vi "TCP Named Service - Server.vi"() -> ()   [LabVIEW 2019]
doc: "创建一个命名服务并在第一个可用端口侦听。当客户端连接该服务时，将发送一个响应字符串至客户端。"
panel:
  in  "服务器关闭":string="服务器VI关闭了连接。"
  in  "停止 2":bool
  out "波形图":dbl[](graph)
  # "概述：演示使用TCP函数初始化可向客户端VI发送数据的命名TCP服务。\n操作步骤:\n1.运行VI。\n2.打开TCP Named Service - Client.vi并按照前面板上的说明操作。\n3.单击停止 停止VI运行。"
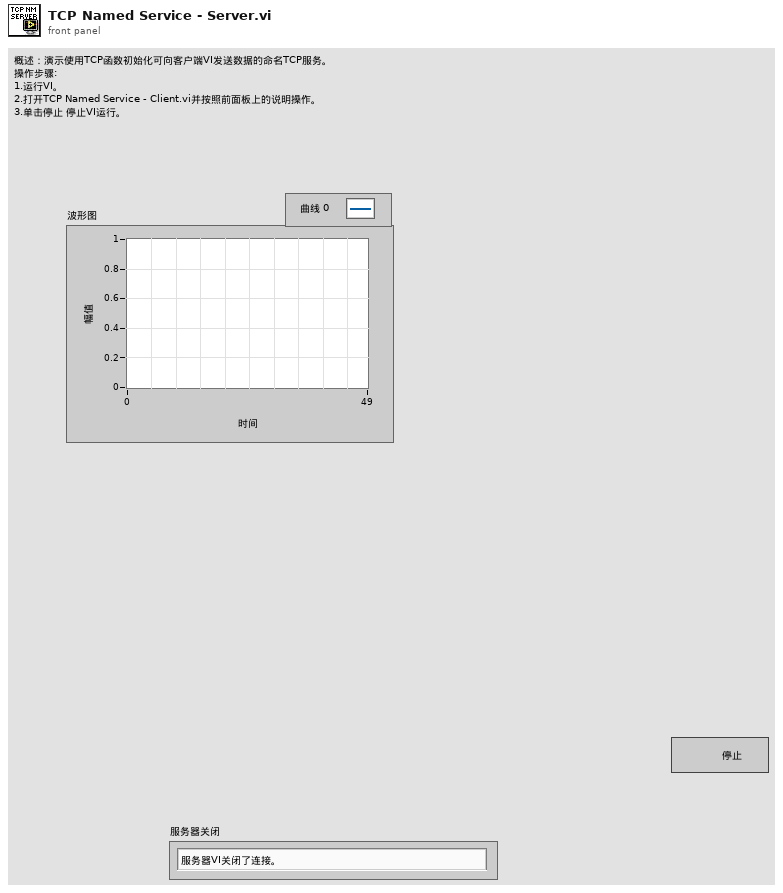
[diagram p1: front panel]
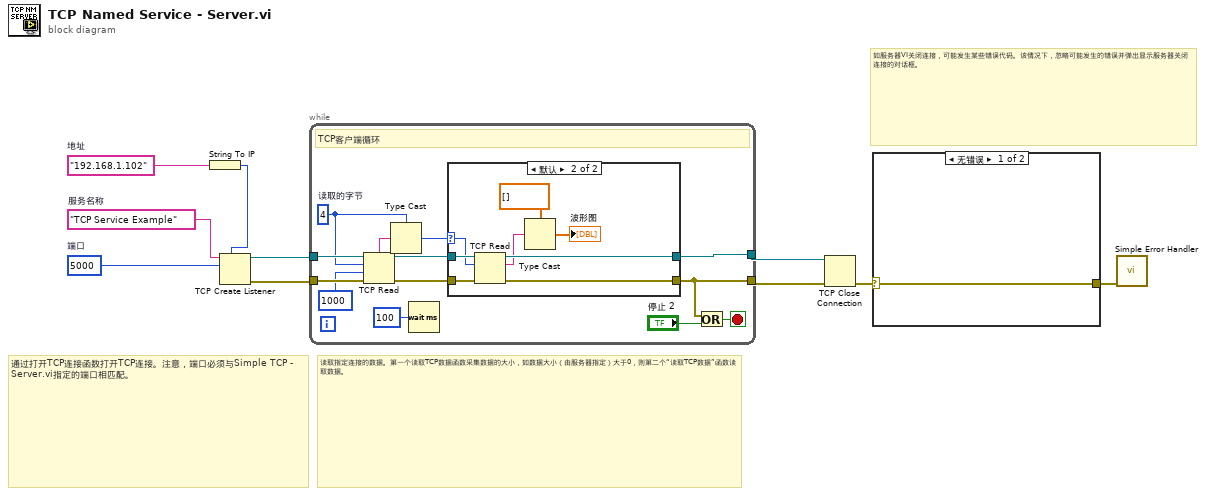
[diagram p0: block diagram]
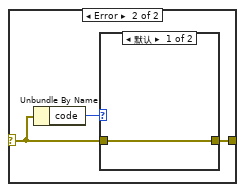
[diagram p2: hidden frame]
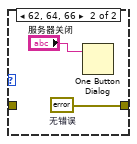
[diagram p3: hidden frame]
diagram:
  w6 = "192.168.1.102"  # 地址
  w8 = u16 5000  # 端口
  w7 = "TCP Service Example"  # 服务名称
  # "如服务器VI关闭连接，可能发生某些错误代码。该情况下，忽略可能发生的错误并弹出显示服务器关闭连接的对话框。"
  # "读取指定连接的数据。第一个读取TCP数据函数采集数据的大小，如数据大小（由服务器指定）大于0，则第二个“读取TCP数据”函数读取数据。"
  # "通过打开TCP连接函数打开TCP连接。注意，端口必须与Simple TCP - Server.vi指定的端口相匹配。"
  n1 = String To IP(1:w6) -> (0:w5:u32)
  n2 = TCP Create Listener(7:w5, 10:w8, 11:w7) -> (0:w3:errorcluster, 3:w4:refnum<k5>)  [unwired: 2 in, 1 out]
  n3 = while {
    tunnel: w3 -> [w19]
    tunnel: w4 -> [w20]
    tunnel: [w14] -> w2
    tunnel: [w13] -> w1
    stop <- w16 stop-if-true
    w18 = 4  # 读取的字节
    # "TCP客户端循环"
    n4 = TCP Read(connection ID=w20, bytes to read=w18, error in (no error)=w19, 9:1000 ("timeout ms (25000)")) -> (connection ID out=w22:refnum<k5>, data out=w23:string, error out=w21:errorcluster)  [unwired: 1 in]
    n5 = Type Cast(type=w18, x=w23) -> (*(type *) &x=w12:i32)
    n6 = Wait (ms)(milliseconds to wait=u32 100) -> ()  [unwired: 1 out]
    n7 = case shown="默认" w12 {
      selector: w12 -> [_ w26]
      tunnel: w22 -> [w25 w33]
      tunnel: w21 -> [w24 w32]
      tunnel: [w25 w29] -> w14
      tunnel: [w24 w28] -> w13
      frame ..0 {
        # "服务器未写入任何数据"
      }
      frame Default {
        n8 = TCP Read(connection ID=w33, bytes to read=w26, error in (no error)=w32) -> (connection ID out=w29:refnum<k5>, data out=w27:string, error out=w28:errorcluster)  [unwired: 2 in]
        n9 = Type Cast(type=dbl[] [] ("chart"), x=w27) -> (*(type *) &x=→"波形图":dbl[])
      }
    }
    n10 = Or(x=w13, y="停止 2") -> (x .or. y?=w16:bool)
  }
  n11 = TCP Close Connection(connection ID=w2, error in (no error)=w1) -> (error out=w10:errorcluster)  [unwired: 1 in, 1 out]
  n12 = case shown="无错误" w10 {
    selector: w10 -> [w34 w36]
    tunnel: [w34 w35] -> w9
    frame No Error {
    }
    frame Error {
      n13 = Unbundle By Name(w36) -> ("code"=w37:i32)
      n14 = case shown="默认" w37 {
        tunnel: w36 -> [w38 _]
        tunnel: [w38 w40] -> w35
        frame Default {
        }
        frame 62, 64, 66 {
          w40 = errorcluster {"status"=FALSE, "code"=0, "source"=""}  # 无错误
          n15 = One Button Dialog(message="服务器关闭") -> ()  [unwired: 1 in, 1 out]
        }
      }
    }
  }
  n16 = call <vilib>:"Simple Error Handler.vi"("error in (no error)"=w9) -> ()  [unwired: 4 in, 5 out]
